vi "KE622x -- Get Arm Layer Params.vi"(0 "Resource In":refnum<visa-resource-name>, 1 "Check For SCPI Errors? (T)":bool=TRUE, 11 "error in (no error)":errorcluster) -> (4 "Resource Out (dupl)":refnum<visa-resource-name>, 8 "Arm Params":T1={"Bypass Arm Layer\nInput Trigger?"=FALSE, "Input Trig Source"=enum."Immediate", "Input Trig Link Line"=enum."1", "Arm Timer Interval (s)"=0.001, "Output Trig Mode"=enum."No Trig Out", "Output Trig Link Line"=enum."1"} {"Arm Timer Interval (s)" min=0.001 max=99999.999 step=0.001 format="%.3f"}, 15 "error out":errorcluster)   [LabVIEW 2010, in "Keithley 622x.lvlib"]
doc: "Returns the parameters for the 'Arm' layer of the trigger model."
uses:
  Keithley 622x.lvlib
  Low Level/Typedefs/KE622x -- Trig Link Line.ctl
  Low Level/Typedefs/KE622x -- Arm Source.ctl
  Low Level/Typedefs/KE622x -- Arm Output Mode.ctl
  Low Level/Typedefs/KE622x -- Arm Timer Interval.ctl
  Typedefs/KE622x -- Arm Layer Params.ctl
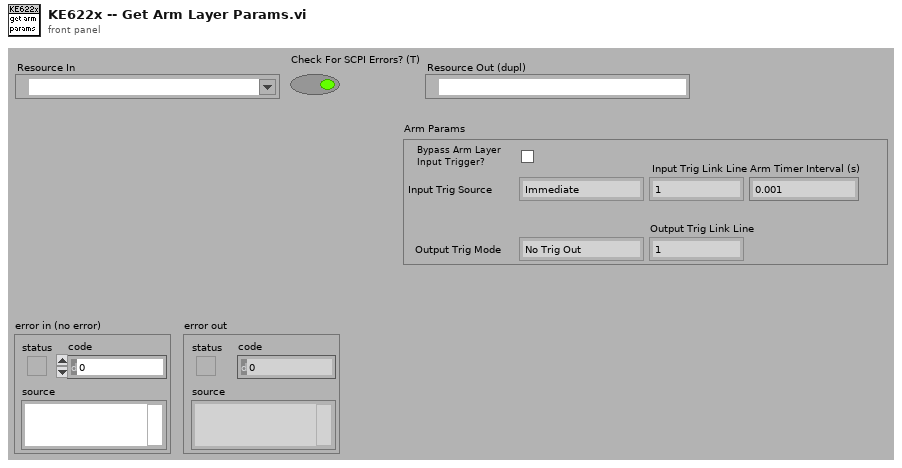
[diagram p1: front panel]
types:
  T1 = typedef "Keithley 622x.lvlib/KE622x -- Arm Layer Params.ctl" = cluster{"Bypass Arm Layer\nInput Trigger?":bool, "Input Trig Source":T2, "Input Trig Link Line":T3, "Arm Timer Interval (s)":T4, "Output Trig Mode":T5, "Output Trig Link Line":T3}
  T2 = typedef "Keithley 622x.lvlib/KE622x -- Arm Source.ctl" = enum16{"Immediate", "Bus (*TRG)", "Timer", "Manual", "Trigger Link", "SOT Falling Edge", "SOT Rising Edge", "SOT Either Edge"}
  T3 = typedef "Keithley 622x.lvlib/KE622x -- Trig Link Line.ctl" = enum16{"1", "2", "3", "4", "5", "6"}
  T4 = typedef "Keithley 622x.lvlib/KE622x -- Arm Timer Interval.ctl" = dbl
  T5 = typedef "Keithley 622x.lvlib/KE622x -- Arm Output Mode.ctl" = enum16{"No Trig Out", "Trig Out On Enter Arm", "Trig Out On Exit Arm"}
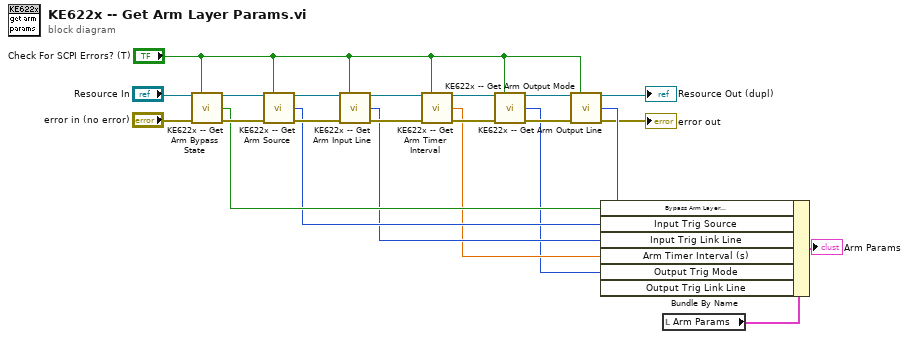
[diagram p0: block diagram]
diagram:
  n1 = call <instrlib>:"KE622x -- Get Arm Bypass State.vi"("Resource In"="Resource In", "Check For SCPI Errors? (T)"="Check For SCPI Errors? (T)", "error in (no error)"="error in (no error)") -> ("Resource Out (dupl)"=w21:refnum<visa-resource-name>, "Arm Layer Bypassed?"=w9:bool, "error out"=w20:errorcluster)  [unwired: 10 in]
  n2 = call "KE622x -- Get Arm Source.vi"("Resource In"=w21, "Check For SCPI Errors? (T)"="Check For SCPI Errors? (T)", "error in (no error)"=w20) -> ("Resource Out (dupl)"=w19:refnum<visa-resource-name>, "Arm Source"=w8:T2, "error out"=w18:errorcluster)  [unwired: 10 in]
  n3 = call <instrlib>:"KE622x -- Get Arm Input Line.vi"("Resource In"=w19, "Check For SCPI Errors? (T)"="Check For SCPI Errors? (T)", "error in (no error)"=w18) -> ("Resource Out (dupl)"=w16:refnum<visa-resource-name>, "Arm Input Line"=w7:T3, "error out"=w17:errorcluster)  [unwired: 10 in]
  n4 = call "KE622x -- Get Arm Timer Interval.vi"("Resource In"=w16, "Check For SCPI Errors? (T)"="Check For SCPI Errors? (T)", "error in (no error)"=w17) -> ("Resource Out (dupl)"=w15:refnum<visa-resource-name>, "Arm Timer Interval (s)"=w6:T4, "error out"=w14:errorcluster)  [unwired: 10 in]
  n5 = call "KE622x -- Get Arm Output Mode.vi"("Resource In"=w15, "Check For SCPI Errors? (T)"="Check For SCPI Errors? (T)", "error in (no error)"=w14) -> ("Resource Out (dupl)"=w12:refnum<visa-resource-name>, "Arm Output Mode"=w5:T5, "error out"=w13:errorcluster)  [unwired: 10 in]
  n6 = call "KE622x -- Get Arm Output Line.vi"("Resource In"=w12, "Check For SCPI Errors? (T)"="Check For SCPI Errors? (T)", "error in (no error)"=w13) -> ("Resource Out (dupl)"=→"Resource Out (dupl)":refnum<visa-resource-name>, "Arm Output Line"=w4:T3, "error out"=→"error out":errorcluster)  [unwired: 10 in]
  n7 = local read "Arm Params"() -> (w10:T1)
  n8 = Bundle By Name(cluster=w10, "Bypass Arm Layer\nInput Trigger?"=w9, "Input Trig Source"=w8, "Input Trig Link Line"=w7, "Arm Timer Interval (s)"=w6, "Output Trig Mode"=w5, "Output Trig Link Line"=w4) -> (→"Arm Params":T1)
